vi "Destroy.vi"(8 "error in (no error)":errorcluster, 11 "ObserverRegistry.lvclass in":refnum<class "ObserverRegistry.lvclass">) -> (0 "error out":errorcluster, 3 "ObserverRegistry.lvclass out":refnum<class "ObserverRegistry.lvclass">)   [LabVIEW 2011, in "Messenging.lvlib" / "ObserverRegistry.lvclass"]
uses:
  ObserverRegistry.lvclass
  ObserverRegistry.lvclass/ObserverRegistry.ctl
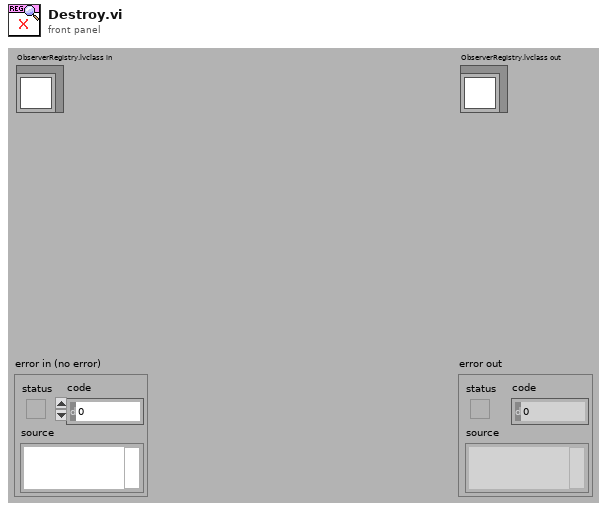
[diagram p1: front panel]
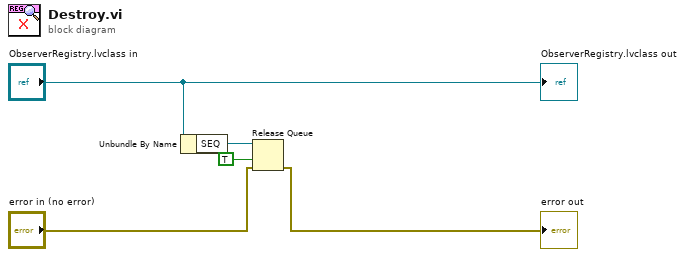
[diagram p0: block diagram]
diagram:
  n1 = Unbundle By Name("ObserverRegistry.lvclass in") -> ("SEQ"=w4:refnum<queue>)
  n2 = Release Queue(queue=w4, force destroy? (F)=TRUE, error in (no error)="error in (no error)") -> (error out=→"error out":errorcluster)  [unwired: 2 out]
  "ObserverRegistry.lvclass out" <- "ObserverRegistry.lvclass in"
